vi "Test-TCP.vi"() -> ()   [LabVIEW 2013, in "MaterialCharacterization.lvlib" / "MC-SM1000.lvclass"]
uses:
  MC-SM1000.lvclass
  Hosts.ctl
  TCP-settings.ctl
panel:
  out "TCP settings":T1={"Target IP"="128.178.146.163", "Target TCP port"=12500, "TCP read mode"=enum."CRLF", "TCP read buffer"=4096, "Read timeout"=5000}
  out "Host in control":T2=enum."Pendant"
  out "Job list":string[](array[string])
  out "Controller temperature":dbl
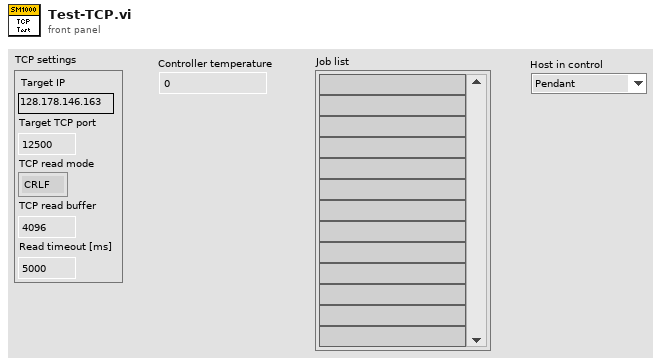
[diagram p1: front panel]
types:
  T1 = typedef "MaterialCharacterization.lvlib/MC-SM1000.lvclass/TCP-settings.ctl" = cluster{"Target IP":string, "Target TCP port":u16, "TCP read mode":enum16{"Standard", "Buffered", "CRLF", "Immediate"}, "TCP read buffer":i32, "Read timeout":i32}
  T2 = typedef "MaterialCharacterization.lvlib/MC-SM1000.lvclass/Hosts.ctl" = enum16{"None", "Pendant", "LANStream", "LAN"}
  T3 = typedef "MaterialCharacterization.lvlib/MC-SM1000.lvclass/Object-reference.ctl" = refnum<data-value>
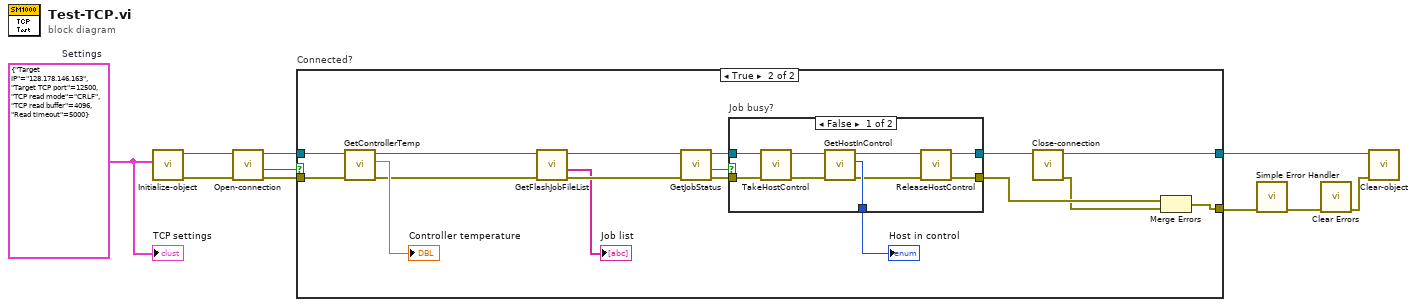
[diagram p0: block diagram]
diagram:
  w10 = T1 {"Target IP"="128.178.146.163", "Target TCP port"=12500, "TCP read mode"=enum."CRLF", "TCP read buffer"=4096, "Read timeout"=5000}  # Settings
  n1 = call "Initialize-object.vi"("TCP settings"=w10) -> ("error out"=w8:errorcluster, "SM1000-control out"=w9:T3)  [unwired: 9 in]
  n2 = call "Open-connection.vi"("error in (no error)"=w8, "SM1000-control in"=w9) -> ("error out"=w6:errorcluster, "Connected?"=w5:bool, "SM1000-control out"=w7:T3)  [unwired: 7 in]
  n3 = case "Connected?" shown="True" w5 {
    tunnel: w7 -> [w11 w29]
    tunnel: w6 -> [w12 w28]
    tunnel: [w12 w18] -> w3
    tunnel: [w11 w13] -> w2
    frame False {
    }
    frame True {
      n4 = call "GetControllerTemp.vi"("error in (no error)"=w28, "SM1000-control in"=w29) -> ("error out"=w15:errorcluster, "Controller temperature"=→"Controller temperature":dbl, "SM1000-control out"=w16:T3)  [unwired: 7 in]
      n5 = call "GetFlashJobFileList.vi"("error in (no error)"=w15, "SM1000-control in"=w16) -> ("error out"=w26:errorcluster, "Job list"=→"Job list":string[], "SM1000-control out"=w27:T3)  [unwired: 7 in]
      n6 = call "GetJobStatus.vi"("error in (no error)"=w26, "SM1000-control in"=w27) -> ("error out"=w23:errorcluster, "Busy?"=w25:bool, "SM1000-control out"=w24:T3)  [unwired: 7 in]
      n7 = case "Job busy?" shown="False" w25 {
        tunnel: w24 -> [w38 w40]
        tunnel: w23 -> [w37 w39]
        tunnel: [w34 _] -> w22
        tunnel: [w31 w40] -> w21
        tunnel: [w30 w39] -> w20
        frame False {
          n8 = call "TakeHostControl.vi"("error in (no error)"=w37, "SM1000-control in"=w38) -> ("error out"=w35:errorcluster, "SM1000-control out"=w36:T3)  [unwired: 8 in]
          n9 = call "GetHostInControl.vi"("error in (no error)"=w35, "SM1000-control in"=w36) -> ("error out"=w32:errorcluster, "Host in control"=w34:T2, "SM1000-control out"=w33:T3)  [unwired: 7 in]
          n10 = call "ReleaseHostControl.vi"("error in (no error)"=w32, "SM1000-control in"=w33) -> ("error out"=w30:errorcluster, "SM1000-control out"=w31:T3)  [unwired: 8 in]
        }
        frame True {
        }
      }
      "Host in control" <- w22
      n11 = call "Close-connection.vi"("SM1000-control in"=w21) -> ("error out"=w19:errorcluster, "SM1000-control out"=w13:T3)  [unwired: 8 in, 1 out]
      n12 = Merge Errors(w20, w19) -> (w18:errorcluster)
    }
  }
  n13 = call <vilib>:"Simple Error Handler.vi"("error in (no error)"=w3) -> ("error out"=w4:errorcluster)  [unwired: 4 in, 4 out]
  n14 = call <vilib>:"Clear Errors.vi"("error in (no error)"=w4) -> ("error out"=w1:errorcluster)  [unwired: 6 in]
  n15 = call "Clear-object.vi"("error in (no error)"=w1, "SM1000-control"=w2) -> ()  [unwired: 8 in, 2 out]
  "TCP settings" <- w10
